vi "waveform_generator_sub.vi"(9 "?":T2={"filter type"=enum."Lowpass", "low cutoff freq"=0.12500000000000006, "high cutoff freq"=0.45000000000000007} {"high cutoff freq" format="%0.2f"; "low cutoff freq" format="%0.4f"}, 10 "Parameters":T3(array[cluster]) {"Signal" items=["Sine", "Square", "Triangle", "Sawtooth"]; "Amplitude" scale=0.0..10.0; "Frequency" scale=0.0..1000.0}, 11 "Filter OFF   Filter ON":bool) -> (3 "Waveform":waveform(dbl))   [LabVIEW 2023]
uses:
  <vilib>/Analysis/3filter.llb/Filter Passband Type.ctl
  <vilib>/Analysis/3filter.llb/Butterworth Filter (DBL).vi
  <vilib>/Analysis/NI_AALBase.lvlib
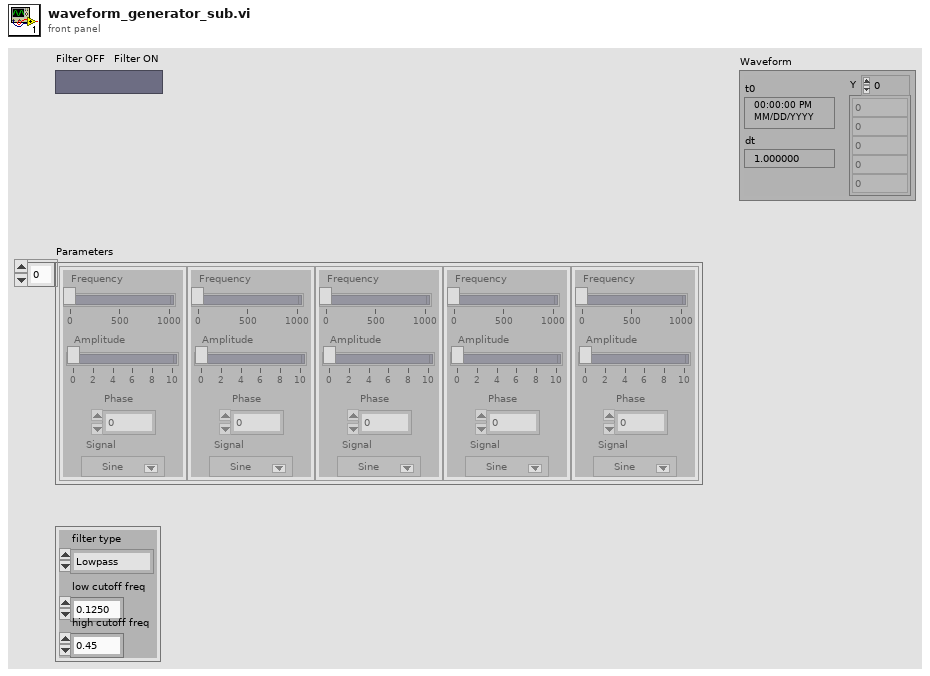
[diagram p1: front panel]
types:
  T1 = typedef "NI_AALBase.lvlib/Filter Passband Type.ctl" = enum32{"Lowpass", "Highpass", "Bandpass", "Bandstop"}
  T2 = cluster{"filter type":T1, "low cutoff freq":dbl, "high cutoff freq":dbl}
  T3 = cluster{"Frequency":dbl, "Amplitude":dbl, "Signal":u16, "Phase":dbl}[]
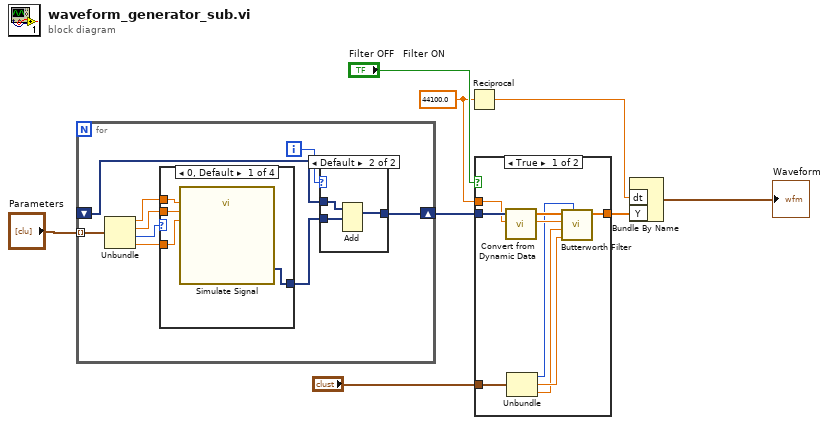
[diagram p0: block diagram]
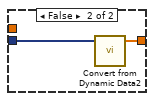
[diagram p2: hidden frame]
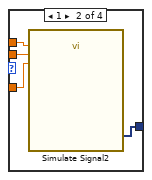
[diagram p3: hidden frame]
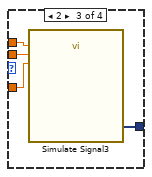
[diagram p4: hidden frame]
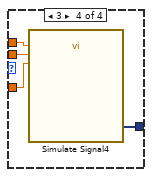
[diagram p5: hidden frame]
diagram:
  w3 = 44100.0
  n1 = for {
    shift-right: [w16] -> w2
    shift-left: _ -> [w15]
    tunnel: "Parameters" -> [w14] mode=indexing
    i -> [w17]
    n2 = Unbundle(w14) -> ("Frequency"=w12:dbl, "Amplitude"=w13:dbl, "Signal"=w11:u16, "Phase"=w9:dbl)
    n3 = case shown="0, Default" w11 {
      tunnel: [w21 w25 w29 w33] -> w10
      tunnel: w13 -> [w20 w24 w28 w32]
      tunnel: w12 -> [w19 w23 w27 w31]
      tunnel: w9 -> [w18 w22 w26 w30]
      frame 0, Default {
        n4 = call "Simulate Signal"("Frequency"=w19, "Amplitude"=w20, "Phase"=w18) -> ("Sine"=w21:dynamicdata)  [unwired: 11 in, 1 out]
      }
      frame 1 {
        n5 = call "Simulate Signal2"("Frequency"=w23, "Amplitude"=w24, "Phase"=w22) -> ("Square"=w25:dynamicdata)  [unwired: 11 in, 1 out]
      }
      frame 2 {
        n6 = call "Simulate Signal3"("Frequency"=w27, "Amplitude"=w28, "Phase"=w26) -> ("Triangle"=w29:dynamicdata)  [unwired: 11 in, 1 out]
      }
      frame 3 {
        n7 = call "Simulate Signal4"("Frequency"=w31, "Amplitude"=w32, "Phase"=w30) -> ("Sawtooth"=w33:dynamicdata)  [unwired: 11 in, 1 out]
      }
    }
    n8 = case shown="Default" w17 {
      tunnel: w10 -> [w34 w37]
      tunnel: [w34 w36] -> w16
      tunnel: w15 -> [_ w35]
      frame 0 {
      }
      frame Default {
        n9 = Add(1:w37, 2:w35) -> (0:w36:dynamicdata)  [unwired: 1 in, 1 out]
      }
    }
  }
  n10 = Reciprocal(x=w3) -> (1/x=w6:dbl)
  n11 = case shown="True" "Filter OFF   Filter ON" {
    tunnel: w2 -> [w45 w47]
    tunnel: [w43 w46] -> w7
    tunnel: w3 -> [w42 _]
    tunnel: "?" -> [w41 _]
    frame True {
      n12 = call "Convert from Dynamic Data"("Dynamic Data Type"=w45) -> ("Array"=w44:dbl[])  [unwired: 3 in]
      n13 = Unbundle(w41) -> ("filter type"=w40:T1, "low cutoff freq"=w39:dbl, "high cutoff freq"=w38:dbl)
      n14 = call-poly <vilib>:"Butterworth Filter.vi"("filter type"=w40, "low cutoff freq: fl"=w39, "high cutoff freq: fh"=w38, "sampling freq: fs"=w42, "X"=w44) -> ("Filtered X"=w43:dbl[])  [unwired: 3 in, 1 out]
    }
    frame False {
      n15 = call "Convert from Dynamic Data2"("Dynamic Data Type"=w47) -> ("Array"=w46:dbl[])  [unwired: 3 in]
    }
  }
  n16 = Bundle By Name("dt"=w6, "Y"=w7) -> (→"Waveform":waveform(dbl))  [unwired: 1 in]
